vi "add channel to configuration.vi"(8 "error in":errorcluster, 10 "TBM channel in":refnum<class "Profibus channel.lvclass">, 11 "Profibus Module configuration in":refnum<class "Profibus Module configuration.lvclass">) -> (0 "error out":errorcluster, 3 "Profibus Module configuration out":refnum<class "Profibus Module configuration.lvclass">)   [LabVIEW 2013, in "Profibus Module configuration.lvclass"]
uses:
  Profibus Module configuration.lvclass
  channel/Profibus channel.lvclass
  <vilib>/NI/Tag Bus/tag/tag descriptor.lvclass/tag descriptor.ctl
  Profibus Module configuration.lvclass/Profibus Module configuration.ctl
  <vilib>/NI/Tag Bus/tag/tag descriptor.lvclass
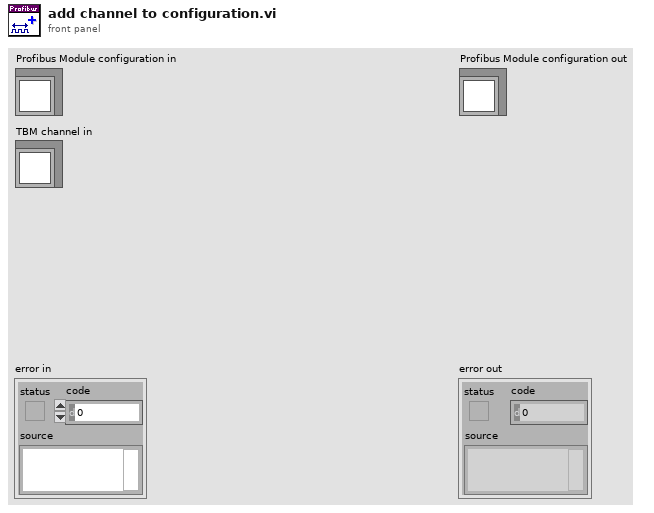
[diagram p1: front panel]
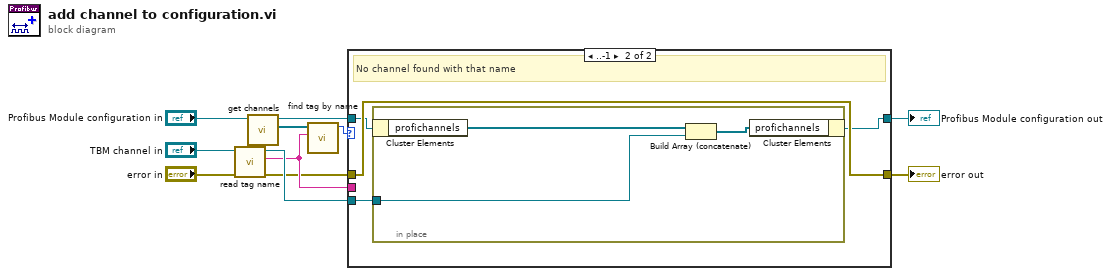
[diagram p0: block diagram]
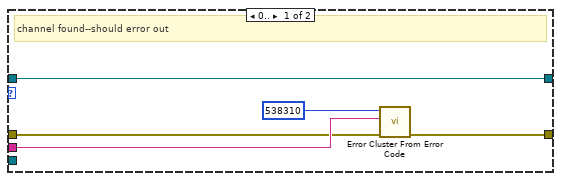
[diagram p2: hidden frame]
diagram:
  n1 = call <vilib>:"read tag name.vi"("error in"="error in", "system tag in"="TBM channel in") -> ("error out"=w2:errorcluster, "name"=w3:string, "system tag out"=w10:refnum<class "Profibus channel.lvclass">)  [unwired: 7 in]
  n2 = call-dynamic "get channels.vi"("Profibus Module configuration in"="Profibus Module configuration in") -> ("channels"=w5:refnum<class "TBM channel.lvclass">[], "Profibus Module configuration out"=w11:refnum<class "Profibus Module configuration.lvclass">)  [unwired: 9 in]
  n3 = call <vilib>:"find tag by name.vi"("name"=w3, "tags in"=w5) -> ("index"=w4:i32)  [unwired: 9 in]
  n4 = case shown="..-1" w4 {
    tunnel: [w16 w19] -> w8
    tunnel: w3 -> [w14 _]
    tunnel: w2 -> [w13 w19]
    tunnel: w11 -> [w12 w18]
    tunnel: w10 -> [_ w20]
    tunnel: [w12 w17] -> w7
    frame 0.. {
      # "channel found--should error out"
      n5 = call <vilib>:"Error Cluster From Error Code.vi"("error in (no error)"=w13, "error message (\"\")"=w14, "error code (0)"=538310) -> ("error out"=w16:errorcluster)  [unwired: 6 in]
    }
    frame ..-1 {
      # "No channel found with that name"
      n6 = in-place {
        in-place-border: w20 -> [w21]
        n7 = in-place-cluster #1(w18) -> ("profichannels"=w22:refnum<class "Profibus channel.lvclass">[])
        n8 = Build Array (concatenate)(w22, w21) -> (w23:refnum<class "Profibus channel.lvclass">[])
        n9 = in-place-cluster #1("profichannels"=w23) -> (w17:refnum<class "Profibus Module configuration.lvclass">)
      }
    }
  }
  "error out" <- w8
  "Profibus Module configuration out" <- w7
